vi "AcquisitionThread.vi"(8 "error in (no error)":errorcluster, 11 "Application Data":T1) -> (0 "error out":errorcluster)   [LabVIEW 2019]
uses:
  Typedefs/#cluster_ApplicationData.ctl
  Typedefs/Acquisition Thread/#cluster_AcqQueueData.ctl
  Typedefs/Acquisition Thread/#enum_AcquisitionTask.ctl
  Typedefs/Saving Thread/#cluster_SavingQueueData.ctl
  Typedefs/Saving Thread/#enum_SavingTask.ctl
  Typedefs/Acquisition Thread/#cluster_AcqThreadData.ctl
  <vilib>/MagicBox/Device/Arduino/Arduino.lvclass
  <vilib>/MagicBox/Peripherals/POX/POX.lvclass
  Typedefs/Acquisition Thread/#enum_AcqThreadState.ctl
  Typedefs/#cluster_GUIRefs.ctl
  LowLevelError.vi
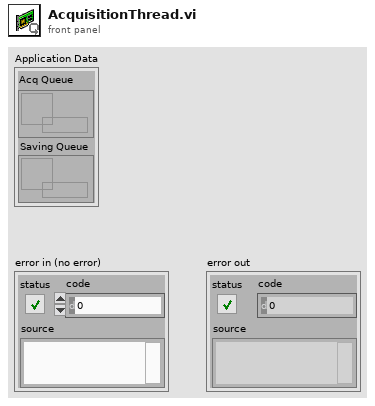
[diagram p1: front panel]
types:
  T1 = typedef "#cluster_ApplicationData.ctl" = cluster{"Acq Queue":refnum<queue>, "Saving Queue":refnum<queue>}
  T2 = typedef "#cluster_AcqThreadData.ctl" = cluster{"Save?":bool, "Arduino":refnum<class "Arduino.lvclass">, "POX":refnum<class "POX.lvclass">, "State":T3, "GUI Refs":T4}
  T3 = typedef "#enum_AcqThreadState.ctl" = enum16{"Idle", "Operate", "Error"}
  T4 = typedef "#cluster_GUIRefs.ctl" = cluster{"Measure":refnum<vi>, "Save?":refnum<vi>, "Stop":refnum<vi>, "Measurement Dir":refnum<vi>, "Heart beat":refnum<vi>, "O2":refnum<vi>, "POX Data History":refnum<vi>}
  T5 = typedef "#cluster_AcqQueueData.ctl" = cluster{"Task":T6, "Data":variant}
  T6 = typedef "#enum_AcquisitionTask.ctl" = enum16{"Init", "Start", "Finish", "Close"}
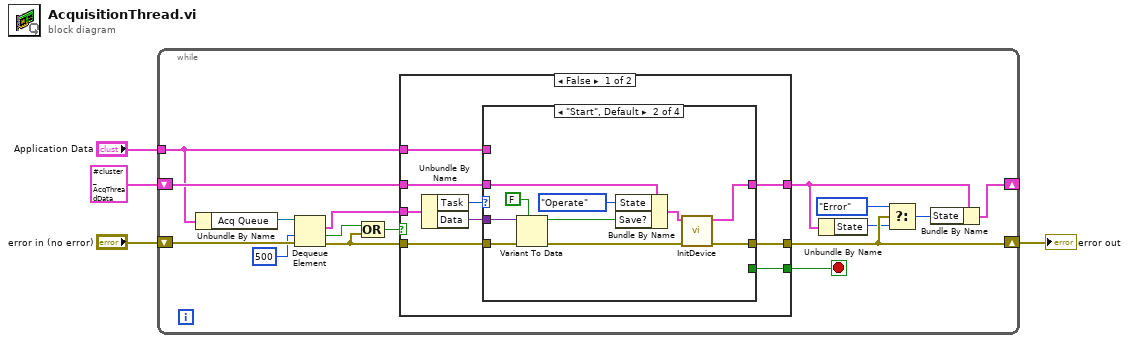
[diagram p0: block diagram]
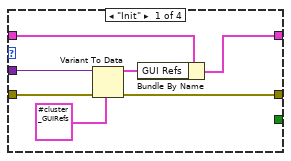
[diagram p2: hidden frame]
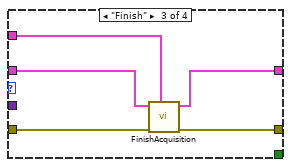
[diagram p3: hidden frame]
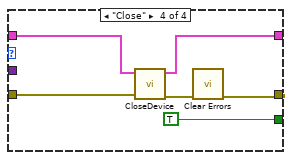
[diagram p4: hidden frame]
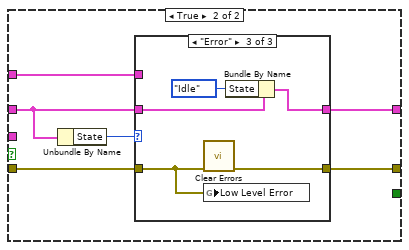
[diagram p5: hidden frame]
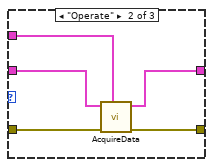
[diagram p7: hidden frame]
diagram:
  n1 = while {
    tunnel: "Application Data" -> [w15]
    shift-right: [w10] -> w2
    shift-left: "error in (no error)" -> [w20]
    shift-right: [w6] -> _
    shift-left: T2 {"Save?"=FALSE, "Arduino"=refnum, "POX"=refnum, "State"=enum."Idle", "GUI Refs"={"Measure"=refnum, "Save?"=refnum, "Stop"=refnum, "Measurement Dir"=refnum, "Heart beat"=refnum, "O2"=refnum, "POX Data History"=refnum}} ("Acq Thread Data") -> [w16]
    stop <- w17 stop-if-true
    n2 = Unbundle By Name(w15) -> ("Acq Queue"=w19:refnum<queue>)
    n3 = Dequeue Element(queue=w19, timeout in ms (-1)=500, error in (no error)=w20) -> (element=w18:T5, timed out?=w13:bool, error out=w11:errorcluster)  [unwired: 1 out]
    n4 = Compound Arithmetic op=OR(w13, w11) -> (w12:bool)
    n5 = case shown="False" w12 {
      tunnel: w18 -> [w29 _]
      tunnel: w11 -> [w26 w63]
      tunnel: [w25 _] -> w17
      tunnel: w16 -> [w24 w61]
      tunnel: [w23 w59] -> w7
      tunnel: w15 -> [w22 w60]
      tunnel: [w21 w58] -> w10
      frame False {
        n6 = Unbundle By Name(w29) -> ("Task"=w28:T6, "Data"=w27:variant)
        n7 = case shown="\"Start\", Default" w28 {
          tunnel: w27 -> [w35 w46 _ _]
          tunnel: w26 -> [w36 w45 w49 w56]
          tunnel: [w31 w41 w50 w54] -> w23
          tunnel: [_ _ _ TRUE] -> w25
          tunnel: w24 -> [w33 w43 w48 w55]
          tunnel: w22 -> [_ _ w47 _]
          tunnel: [w30 w38 w51 w52] -> w21
          frame "Init" {
            n8 = Variant To Data(error in=w36, type=T4 {"Measure"=refnum, "Save?"=refnum, "Stop"=refnum, "Measurement Dir"=refnum, "Heart beat"=refnum, "O2"=refnum, "POX Data History"=refnum} ("GUI Refs"), Variant=w35) -> (data=w32:T4, error out=w30:errorcluster)
            n9 = Bundle By Name(cluster=w33, "GUI Refs"=w32) -> (w31:T2)
          }
          frame "Start", Default {
            n10 = Variant To Data(error in=w45, type=FALSE, Variant=w46) -> (data=w42:bool, error out=w39:errorcluster)
            n11 = Bundle By Name(cluster=w43, "State"=#enum_AcqThreadState."Operate", "Save?"=w42) -> (w40:T2)
            n12 = call "InitDevice.vi"("error in (no error)"=w39, "Acq Thread Data in"=w40) -> ("error out"=w38:errorcluster, "Acq Thread Data out"=w41:T2)  [unwired: 8 in]
          }
          frame "Finish" {
            n13 = call "FinishAcquisition.vi"("Application Data"=w47, "error in (no error)"=w49, "Acq Thread Data"=w48) -> ("error out"=w51:errorcluster, "Acq Thread Data out"=w50:T2)  [unwired: 7 in]
          }
          frame "Close" {
            n14 = call "CloseDevice.vi"("error in (no error)"=w56, "Acq Thread Data in"=w55) -> ("error out"=w53:errorcluster, "Acq Thread Data out"=w54:T2)  [unwired: 8 in]
            n15 = call <vilib>:"Clear Errors.vi"("error in (no error)"=w53) -> ("error out"=w52:errorcluster)  [unwired: 5 in, 1 out]
          }
        }
      }
      frame True {
        n16 = Unbundle By Name(w61) -> ("State"=w62:T3)
        n17 = case shown="\"Error\"" w62 {
          tunnel: w63 -> [w64 w70 w71]
          tunnel: w61 -> [w65 w67 w74]
          tunnel: [w64 w66 w75] -> w58
          tunnel: w60 -> [_ w68 _]
          tunnel: [w65 w69 w73] -> w59
          frame "Idle", Default {
          }
          frame "Operate" {
            n18 = call "AcquireData.vi"("Application Data"=w68, "error in (no error)"=w70, "Acq Thread Data in"=w67) -> ("error out"=w66:errorcluster, "Acq Thread Data out"=w69:T2)  [unwired: 7 in]
          }
          frame "Error" {
            n19 = call <vilib>:"Clear Errors.vi"("error in (no error)"=w71) -> ("error out"=w75:errorcluster)  [unwired: 5 in, 1 out]
            n20 = global write "LowLevelError.vi" "Low Level Error"(w71) -> ()
            n21 = Bundle By Name(cluster=w74, "State"=#enum_AcqThreadState."Idle") -> (w73:T2)
          }
        }
      }
    }
    n22 = Unbundle By Name(w7) -> ("State"=w9:T3)
    n23 = Select(t=#enum_AcqThreadState."Error", s=w10, f=w9) -> (s? t:f=w5:T3)
    n24 = Bundle By Name(cluster=w7, "State"=w5) -> (w6:T2)
  }
  "error out" <- w2
